vi "DSF.Engine.Framework.Initialize.Transfers.vi"(8 "error in (no error)":errorcluster, 11 "Framework in":refnum<class "Framework.lvclass">) -> (0 "error out":errorcluster, 2 "All Transfers":refnum<class "DSF.Engine.Transfer.lvclass">[](array[class]), 3 "Framework out":refnum<class "Framework.lvclass">)   [LabVIEW 2017, in "DSF.Engine.lvlib" / "Framework.lvclass"]
uses:
  Framework.lvclass
  Transfer/DSF.Engine.Transfer.lvclass
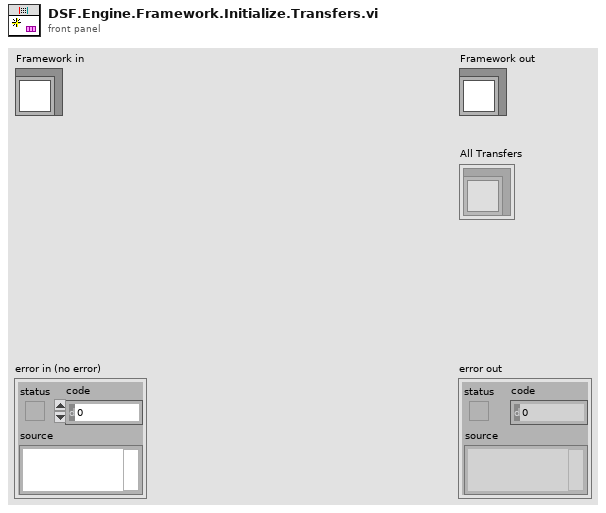
[diagram p1: front panel]
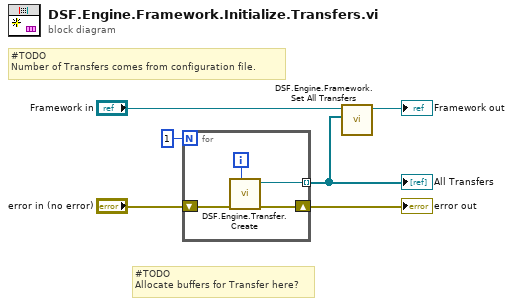
[diagram p0: block diagram]
diagram:
  # "#TODO\nAllocate buffers for Transfer here?"
  # "#TODO\nNumber of Transfers comes from configuration file."
  n1 = for {
    N: 1 -> [_]
    shift-right: [w9] -> w5
    shift-left: "error in (no error)" -> [w10]
    tunnel: [w8] -> w1 mode=indexing
    i -> [w7]
    n2 = call "DSF.Engine.Transfer.Create.vi"("id"=w7, "error in (no error)"=w10) -> ("error out"=w9:errorcluster, "Transfer out"=w8:refnum<class "DSF.Engine.Transfer.lvclass">)  [unwired: 8 in]
  }
  "error out" <- w5
  "All Transfers" <- w1
  n3 = call "DSF.Engine.Framework.Set All Transfers.vi"("All Transfers"=w1, "Framework in"="Framework in") -> ("Framework out"=→"Framework out":refnum<class "Framework.lvclass">)  [unwired: 9 in]
